vi "niRFUtil MEAS Compute Waveform RMS.vi"(7 "Waveform In":T2 {"y" format="%.2f"; "dx" format="%^.2e"; "x0" format="%^.2e"}, 13 "Burst Present":T1) -> (3 "RMS (V)":sgl format="%#.2f", 8 "Waveform Out":T2 {"y" format="%.2f"; "dx" format="%^.2e"; "x0" format="%^.2e"}, 10 "Burst Positions":cluster{"Start (s)":dbl, "Duration (s)":dbl}[](array[cluster]) {"Start (s)" format="%^.3e"; "Duration (s)" format="%^.3e"})   [LabVIEW 2015, in "niRFUtil.lvlib"]
doc: "(c) Copyright 2006, National Instruments, Inc. This VI may not be duplicated, sold, or distributed without written consent from National Instruments."
uses:
  niRFUtil.lvlib
  Includes/niRFUtil INC Complex Waveform.ctl
  Includes/niRFUtil INC Complex Array.ctl
  Includes/niRFUtil INC Burst Present.ctl
  Includes/niRFUtil INC Edge Detection Settings.ctl
  Includes/niRFUtil INC Edge Type.ctl
  Waveform Manipulation/niRFUtil WFM Concatenate Waveforms (complex wfm).vi
  Waveform Manipulation/niRFUtil WFM Parse Waveform - Duration (complex wfm).vi
  Waveform Manipulation/niRFUtil WFM Detect Multiple Bursts (complex wfm).vi
  Waveform Manipulation/niRFUtil WFM Detect Edge (complex wfm).vi
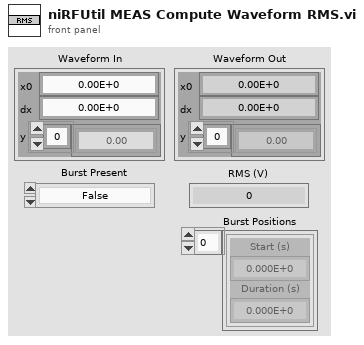
[diagram p1: front panel]
types:
  T1 = typedef "niRFUtil.lvlib/niRFUtil INC Burst Present.ctl" = enum16{"False", "True", "Multiple Bursts"}
  T2 = typedef "niRFUtil.lvlib/niRFUtil INC Complex Waveform.ctl" = cluster{"x0":dbl, "dx":dbl, "y":T3}
  T3 = typedef "niRFUtil.lvlib/niRFUtil INC Complex Array.ctl" = csg[]
  T4 = typedef "niRFUtil.lvlib/niRFUtil INC Edge Detection Settings.ctl" = cluster{"Mode":enum16{"Sliding Window", "Threshold"}, "Sliding Window Settings":cluster{"Chunks":i32, "Threshold (dB)":dbl}, "Threshold Settings":cluster{"Threshold Level (dB)":dbl, "Minimum Quiet Time (s)":dbl, "Threshold Type":enum16{"Relative", "Absolute"}}}
  T5 = typedef "niRFUtil.lvlib/niRFUtil INC Edge Type.ctl" = enum16{"Rising", "Falling"}
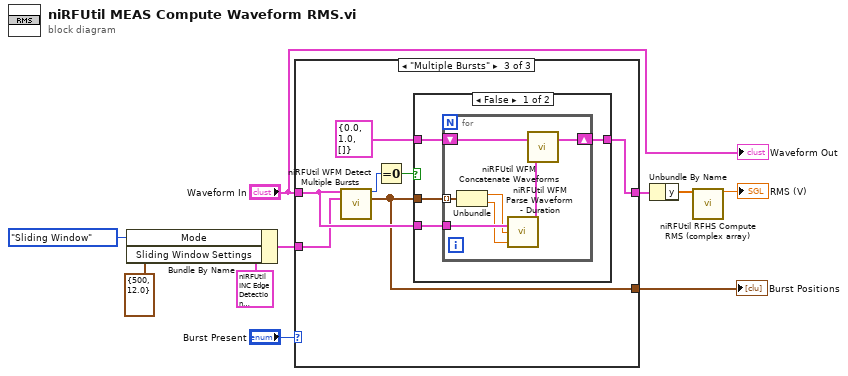
[diagram p0: block diagram]
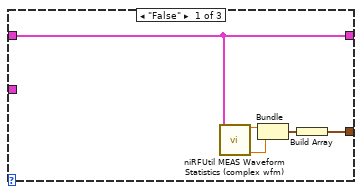
[diagram p2: hidden frame]
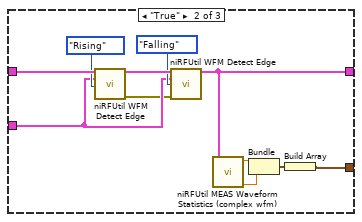
[diagram p3: hidden frame]
diagram:
  n1 = Bundle By Name(cluster=T4 {"Mode"=enum."Sliding Window", "Sliding Window Settings"={"Chunks"=500, "Threshold (dB)"=12.0}, "Threshold Settings"={"Threshold Level (dB)"=-50.0, "Minimum Quiet Time (s)"=0.0001, "Threshold Type"=enum."Absolute"}} ("Burst Detection Settings"), "Mode"=enum16{"Sliding Window", "Threshold"}."Sliding Window", "Sliding Window Settings"=cluster{"Chunks":i32, "Threshold (dB)":dbl} {"Chunks"=500, "Threshold (dB)"=12.0}) -> (w6:T4)
  n2 = case shown="\"Multiple Bursts\"" "Burst Present" {
    tunnel: "Waveform In" -> [w13 w26 w33]
    tunnel: w6 -> [_ w22 w30]
    tunnel: [w13 w18 w29] -> w8
    tunnel: [w14 w19 w28] -> w7
    frame "False" {
      n3 = call "niRFUtil MEAS Waveform Statistics (complex wfm).vi"("Waveform In"=w13) -> ("Start"=w12:dbl, "Duration"=w11:dbl)  [unwired: 4 in, 2 out]
      n4 = Bundle("Start"=w12, "Duration"=w11) -> (w15:cluster{"Start":dbl, "Duration":dbl})  [unwired: 1 in]
      n5 = Build Array(w15) -> (w14:cluster{"Start":dbl, "Duration":dbl}[])
    }
    frame "True" {
      n6 = call-poly "niRFUtil WFM Detect Edge.vi"("Input Waveform"=w26, "Edge Detection Settings"=w22, "Edge Type"=niRFUtil_INC_Edge_Type."Rising") -> ("Output Waveform"=w24:T2, "error out"=w21:errorcluster)  [unwired: 9 in, 2 out]
      n7 = call-poly "niRFUtil WFM Detect Edge.vi"("Input Waveform"=w24, "Edge Detection Settings"=w22, "Edge Type"=niRFUtil_INC_Edge_Type."Falling", "error in (no error)"=w21) -> ("Output Waveform"=w18:T2)  [unwired: 8 in, 3 out]
      n8 = call "niRFUtil MEAS Waveform Statistics (complex wfm).vi"("Waveform In"=w18) -> ("Start"=w17:dbl, "Duration"=w16:dbl)  [unwired: 4 in, 2 out]
      n9 = Bundle("Start"=w17, "Duration"=w16) -> (w20:cluster{"Start":dbl, "Duration":dbl})  [unwired: 1 in]
      n10 = Build Array(w20) -> (w19:cluster{"Start":dbl, "Duration":dbl}[])
    }
    frame "Multiple Bursts" {
      n11 = call-poly "niRFUtil WFM Detect Multiple Bursts.vi"("Waveform In (Ohm Voltage)"=w33, "Burst Detection Settings"=w30) -> ("Number of Bursts Detected"=w31:i32, "Burst Positions"=w28:cluster{"Start (s)":dbl, "Duration (s)":dbl}[])  [unwired: 12 in]
      n12 = Equal To 0?(x=w31) -> (x = 0?=w32:bool)
      n13 = case shown="False" w32 {
        tunnel: w28 -> [w37 _]
        tunnel: w33 -> [w36 w45]
        tunnel: [w35 w45] -> w29
        tunnel: T2 {"x0"=0.0, "dx"=1.0, "y"=[]} ("Waveform Constant") -> [w34 _]
        frame False {
          n14 = for {
            tunnel: w37 -> [w43] mode=indexing
            tunnel: w36 -> [w44]
            shift-right: [w38] -> w35
            shift-left: w34 -> [w40]
            n15 = Unbundle(w43) -> ("Start (s)"=w42:dbl, "Duration (s)"=w41:dbl)
            n16 = call-poly "niRFUtil WFM Parse Waveform - Duration.vi"("Duration (Inf)"=w41, "Start (-Inf)"=w42, "Waveform In"=w44) -> ("Waveform Out"=w39:T2)  [unwired: 2 in]
            n17 = call-poly "niRFUtil WFM Concatenate Waveforms.vi"("Waveform 2 In"=w39, "Waveform 1 In"=w40) -> ("Waveform Out"=w38:T2)  [unwired: 1 in]
          }
        }
        frame True {
        }
      }
    }
  }
  "Burst Positions" <- w7
  n18 = Unbundle By Name(w8) -> ("y"=w2:T3)
  n19 = call "niRFUtil RFHS Compute RMS (complex array).vi"("Complex Array (V)"=w2) -> ("RMS (V)"=→"RMS (V)":sgl)  [unwired: 14 in]
  "Waveform Out" <- "Waveform In"
